vi "demo target.vi"() -> ()   [LabVIEW 2025]
panel:
  out "P (bar)":dbl
  in  "V11":bool
  in  "V10":bool
  in  "V9":bool
  in  "V8":bool
  in  "V7":bool
  in  "V6c":bool
  in  "V6b":bool
  in  "V6a":bool
  in  "V5c":bool
  in  "V5b":bool
  in  "V5a":bool
  in  "V4":bool
  in  "V3":bool
  in  "MFC-3":dbl
  in  "MFC-2":dbl
  in  "MFC-1":dbl
  in  "stop":bool
  in  "Time Stamp":timestamp
  in  "Tab Control":enum32{"Page 1", "Page 2"}(tab)
  in  "String on a page":string
  in  "Boolean on a page":bool
  in  "Numeric on a page":dbl
  in  "Tab Control 2":enum32{"Page 1", "Page 2"}(tab)
  in  "Numeric far away":dbl
  in  "Cluster":T1
  in  "String Array":string[](array[string])=["", "", "", "", ""]
  in  "Boolean Array":bool[](array[boolean])=[FALSE, FALSE, FALSE, FALSE, FALSE]
  in  "Numeric Array":dbl[](array[numeric])=[0.0, 0.0, 0.0, 0.0, 0.0]
  out "String 2":string
  out "Boolean 2":bool
  out "Numeric 2":dbl
  in  "String":string
  in  "Boolean":bool
  in  "Numeric":dbl
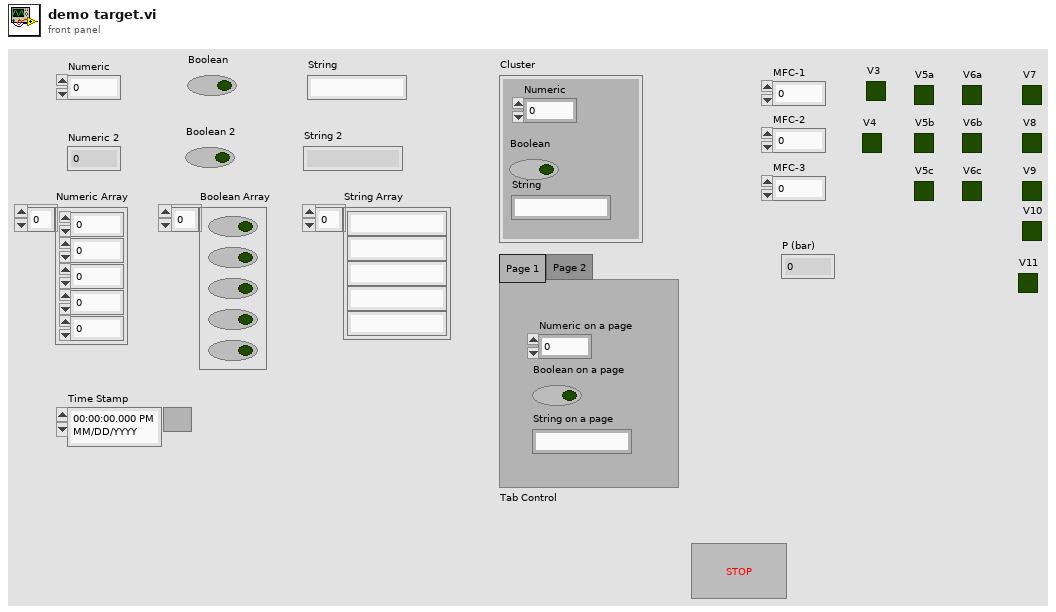
[diagram p1: front panel]
types:
  T1 = cluster{"Numeric":dbl, "Boolean":bool, "String":string}
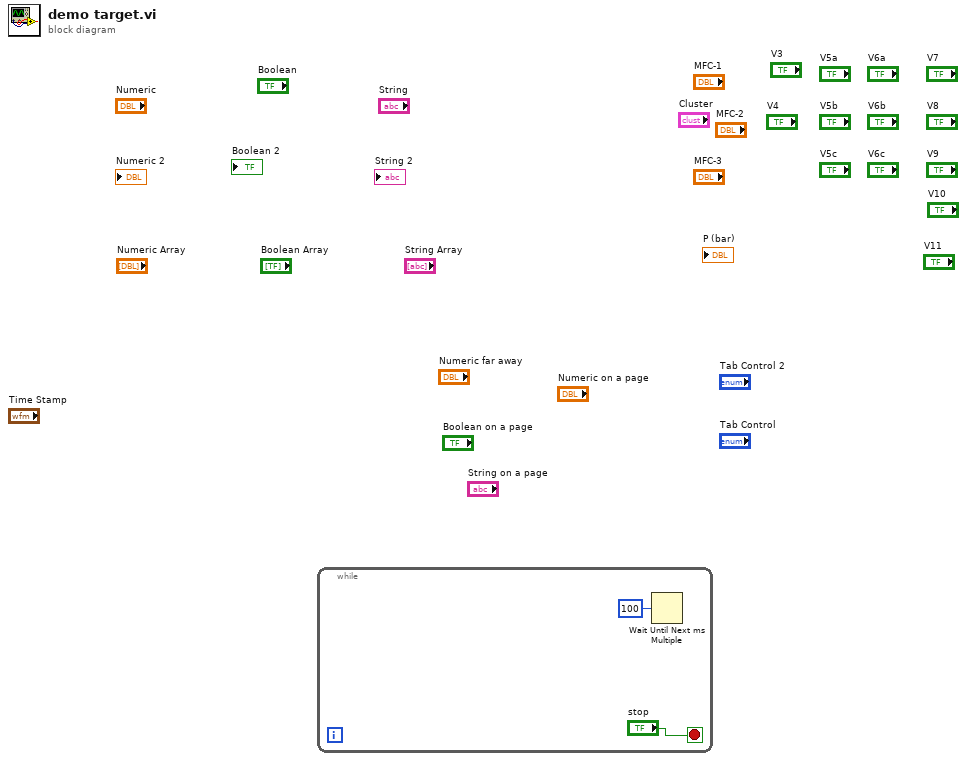
[diagram p0: block diagram]
diagram:
  n1 = while {
    stop <- "stop" stop-if-true
    n2 = Wait Until Next ms Multiple(millisecond multiple=u32 100) -> ()  [unwired: 1 out]
  }
